vi "initialize.vi"(0 "HGF_NetworkEvent":refnum<class "HGF_NetworkEvent.lvclass">, 3 "initializationData":variant, 5 "error in (no error)":errorcluster, 7 "binaryString":string, 8 "I8 Array":i8[](array[numeric]), 9 "prependSize? (T)":bool, 11 "byteOrder (0:big-endian, network order)":T1(ring)) -> (14 "dup HGF_NetworkEvent":refnum<class "HGF_NetworkEvent.lvclass">, 17 "found?":bool, 19 "error out":errorcluster)   [LabVIEW 2014, in "HGF_BaseClasses.lvlib" / "HGF_NetworkEvent.lvclass"]
doc: "This is a dynamic dispatch VI to be implemented by child classes to initialize their attributes.\n\n<B>Recommendation:</B> Use Variant for initialization data."
uses:
  HGF_NetworkEvent.lvclass
  HGF_TriggeredEvent/HGF_TriggeredEvent.lvclass
  HGF_NetworkVisitor/HGF_NetworkVisitor.lvclass
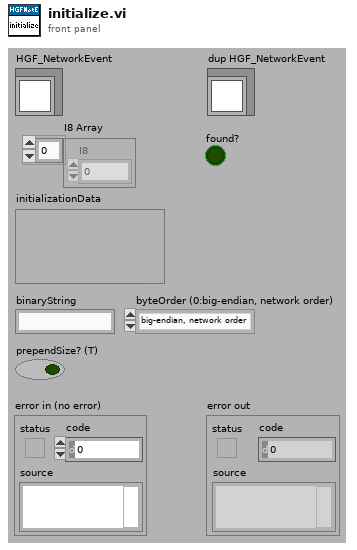
[diagram p1: front panel]
types:
  T1 = enum16{"big-endian, network order", "native, host order", "little-endian"}
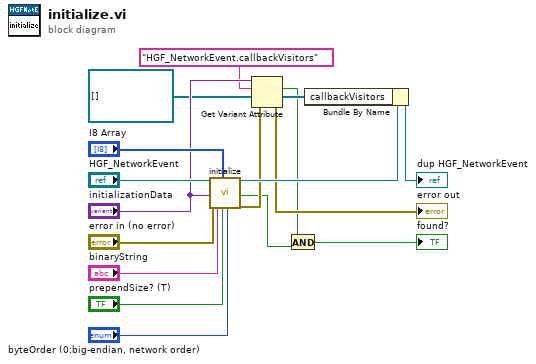
[diagram p0: block diagram]
diagram:
  n1 = call-parent "initialize.vi"("HGF_Timing"="HGF_NetworkEvent", "initializationData"="initializationData", "error in (no error)"="error in (no error)", "binaryString"="binaryString", "I8 Array"="I8 Array", "prependSize? (T)"="prependSize? (T)", "byteOrder (0:big-endian, network order)"="byteOrder (0:big-endian, network order)") -> ("dup HGF_Timing"=w11:refnum<class "HGF_NetworkEvent.lvclass">, "found?"=w2:bool, "error out"=w6:errorcluster)  [unwired: 10 out]
  n2 = Get Variant Attribute(Variant="initializationData", name="HGF_NetworkEvent.callbackVisitors", default value (empty Variant)=refnum<class "HGF_NetworkVisitor.lvclass">[] [] ("callbackVisitors"), error in=w6) -> (found=w3:bool, value=w4:refnum<class "HGF_NetworkVisitor.lvclass">[], error out=→"error out":errorcluster)  [unwired: 1 out]
  n3 = And(x=w3, y=w2) -> (x .and. y?=→"found?":bool)
  n4 = Bundle By Name(cluster=w11, "callbackVisitors"=w4) -> (→"dup HGF_NetworkEvent":refnum<class "HGF_NetworkEvent.lvclass">)
